vi "Get Family.vi"(8 "error in (no error)":errorcluster, 11 "DOM document in":refnum<k20>) -> (0 "error out":errorcluster, 2 "family":T1, 3 "DOM document out":refnum<k20>)   [LabVIEW 2017, in "Error File Management.lvlib"]
uses:
  Error File Management.lvlib
  Controls/NI Family.ctl
  <vilib>/xml/Close Reference(Node).vi
  <vilib>/xml/NI_XML.lvlib
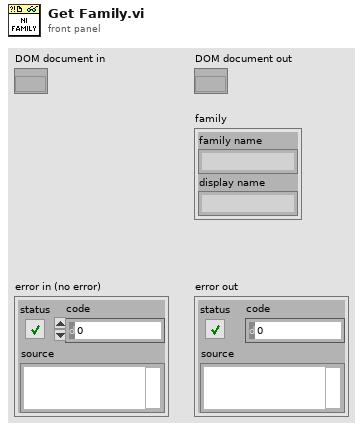
[diagram p1: front panel]
types:
  T1 = typedef "Error File Management.lvlib/NI Family.ctl" = cluster{"family name":string, "display name":string}
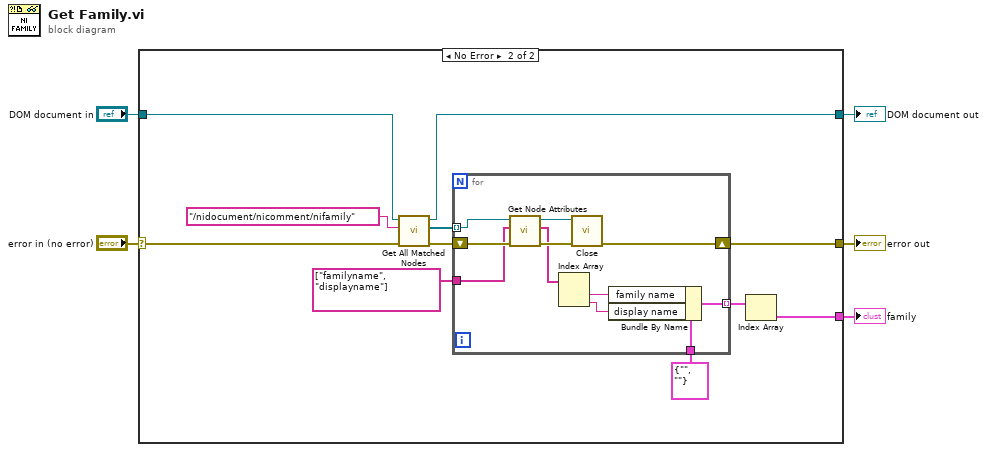
[diagram p0: block diagram]
diagram:
  n1 = case shown="No Error" "error in (no error)" {
    selector: "error in (no error)" -> [w7 w15]
    tunnel: [w6 w18] -> w5
    tunnel: "DOM document in" -> [w6 w17]
    tunnel: [w7 w10] -> w2
    tunnel: [_ w9] -> w1
    frame Error {
    }
    frame No Error {
      n2 = call <vilib>:"Get All Matched Nodes.vi"("error in (no error)"=w15, "XPath expression"="/nidocument/nicomment/nifamily", "node in"=w17) -> ("error out"=w13:errorcluster, "node result array"=w12:refnum<k20>[], "node out"=w18:refnum<k20>)  [unwired: 6 in]
      n3 = for {
        tunnel: w12 -> [w28] mode=indexing
        shift-right: [w29] -> w10
        shift-left: w13 -> [w27]
        tunnel: string[] ["familyname", "displayname"] -> [w26]
        tunnel: [w20] -> w11 mode=indexing
        tunnel: T1 {"family name"="", "display name"=""} ("family") -> [w19]
        n4 = call "Get Node Attributes.vi"("error in (no error)"=w27, "names"=w26, "node in"=w28) -> ("error out"=w25:errorcluster, "values"=w23:string[], "node out"=w24:refnum<k20>)  [unwired: 6 in]
        n5 = Index Array(array=w23) -> (element #1=w22:string, element #2=w21:string)  [unwired: 2 in]
        n6 = call-poly <vilib>:"Close.vi"("error in (no error)"=w25, "node"=w24) -> ("error out"=w29:errorcluster)  [unwired: 7 out]
        n7 = Bundle By Name(cluster=w19, "family name"=w22, "display name"=w21) -> (w20:T1)
      }
      n8 = Index Array(array=w11) -> (element=w9:T1)  [unwired: 1 in]
    }
  }
  "DOM document out" <- w5
  "error out" <- w2
  "family" <- w1
